vi "test_GetPublicEvents_SMO.vi"(8 "error in (no error)":errorcluster, 11 "TestCase in":refnum<class "SMO_TestCase.lvclass">) -> (0 "error out":errorcluster, 3 "TestCase out":refnum<class "SMO_TestCase.lvclass">)   [LabVIEW 2013, in "SMO_TestCase.lvclass"]
uses:
  SMO_TestCase.lvclass
  SMO_TestCase.lvclass/SMO_TestCase.ctl
  <vilib>/addons/_JKI Toolkits/VI Tester/TestCase.llb/TestCase.lvclass
  Projects/JKI SMO Git/JKI-State-Machine-Objects/src/SMO/SMO.lvclass
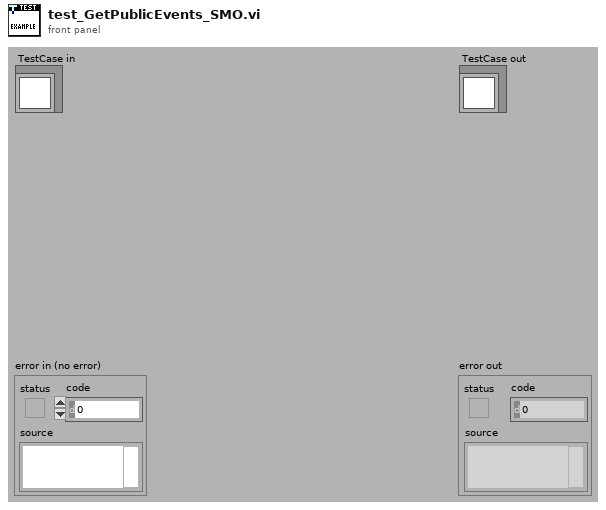
[diagram p1: front panel]
types:
  T1 = typedef "SMO.lvclass/Public Events.ctl" = cluster{"Error":refnum<user-event>}
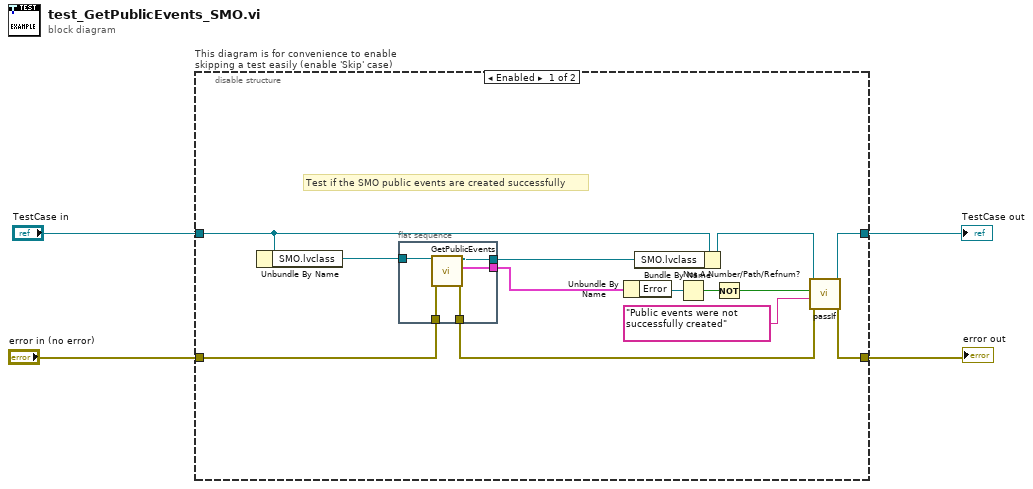
[diagram p0: block diagram]
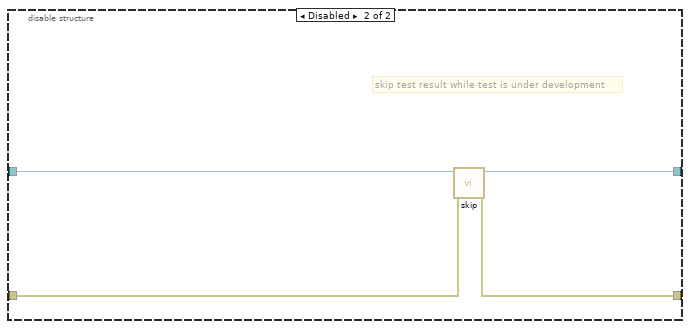
[diagram p2: hidden frame]
diagram:
  n1 = disable-structure "This diagram is for convenience to enable skipping a test easily (enable 'Skip' case)" shown="Enabled" {
    disable-tunnel: "TestCase in" -> [w15 w26]
    disable-tunnel: [w6 w24] -> w1
    disable-tunnel: [w8 w25] -> w3
    disable-tunnel: "error in (no error)" -> [w16 w23]
    frame Enabled {
      # "Test if the SMO public events are created successfully"
      n2 = Unbundle By Name(w15) -> ("SMO.lvclass"=w17:refnum<class "SMO.lvclass">)
      n3 = flat-sequence {
        tunnel: w17 -> [w22]
        tunnel: w16 -> [w21]
        tunnel: [w20] -> w14
        tunnel: [w19] -> w13
        tunnel: [w18] -> w9
        frame #0 {
          n4 = call "GetPublicEvents.vi"("error in (no error)"=w21, "SMO"=w22) -> ("error out"=w18:errorcluster, "Public Events"=w19:T1, "SMO out"=w20:refnum<class "SMO.lvclass">)  [unwired: 7 in]
        }
      }
      n5 = Unbundle By Name(w13) -> ("Error"=w12:refnum<user-event>)
      n6 = Bundle By Name(cluster=w15, "SMO.lvclass"=w14) -> (w7:refnum<class "SMO_TestCase.lvclass">)
      n7 = Not A Number/Path/Refnum?(number/path/refnum=w12) -> (NaN/Path/Refnum?=w11:bool)
      n8 = Not(x=w11) -> (.not. x?=w10:bool)
      n9 = call-dynamic "passIf.vi"("error in (no error)"=w9, "message (\"\")"="Public events were not successfully created" ("message (\"\")"), "pass"=w10, "TestCase in"=w7) -> ("error out"=w8:errorcluster, "TestCase out"=w6:refnum<class "SMO_TestCase.lvclass">)  [unwired: 6 in]
    }
    frame Disabled {
      # "skip test result while test is under development"
      n10 = call <vilib>:"skip.vi"("error in (no error)"=w23, "TestCase in"=w26) -> ("error out"=w25:errorcluster, "TestCase out"=w24:refnum<class "SMO_TestCase.lvclass">)  [unwired: 8 in]
    }
  }
  "error out" <- w3
  "TestCase out" <- w1
